vi "Thermopower-v2-SMU1ar-withnVmeter.vi"(0 "Gate Start":dbl format="%#_13g", 1 "hold time (sec)":dbl=10.0 format="%#_13g", 2 "Gate step - extra milliseconds to wait":u32=20000, 4 "N Gate Intervals":i32=7, 5 "Gate Step":dbl=-6.0, 6 "N Heater Intervals":i32=7, 7 "Heater Step":dbl=3.3) -> ()   [LabVIEW 2016]
uses:
  Driver/New driver/Agilent 415X Series.lvlib
  <vilib>/Utility/file.llb/Write To Spreadsheet File (DBL).vi
  <vilib>/Utility/file.llb/Read From Spreadsheet File (DBL).vi
panel:
  out "Voltage across heater (VSU 1 and SMU4) 2":dbl[][](graph)
  out "error out 2":errorcluster
  out "Gate Voltage (SMU 3) 2":dbl[](graph)
  out "Thermal Voltage (SMU2), SMU1 is Common 2":dbl[](graph)
  out "SPA VISA resource name 2":refnum<visa-resource-name>
  out "Voltage across heater (VSU 1 and SMU4)":dbl[][](graph)
  out "Gate Voltage (SMU 3)":dbl[](graph)
  out "Thermal Voltage (SMU2), SMU1 is Common":dbl[](graph)
  in  "SPA VISA resource name":refnum<visa-resource-name>="GPIB0::14::INSTR"
  in  "error in (no error)":errorcluster
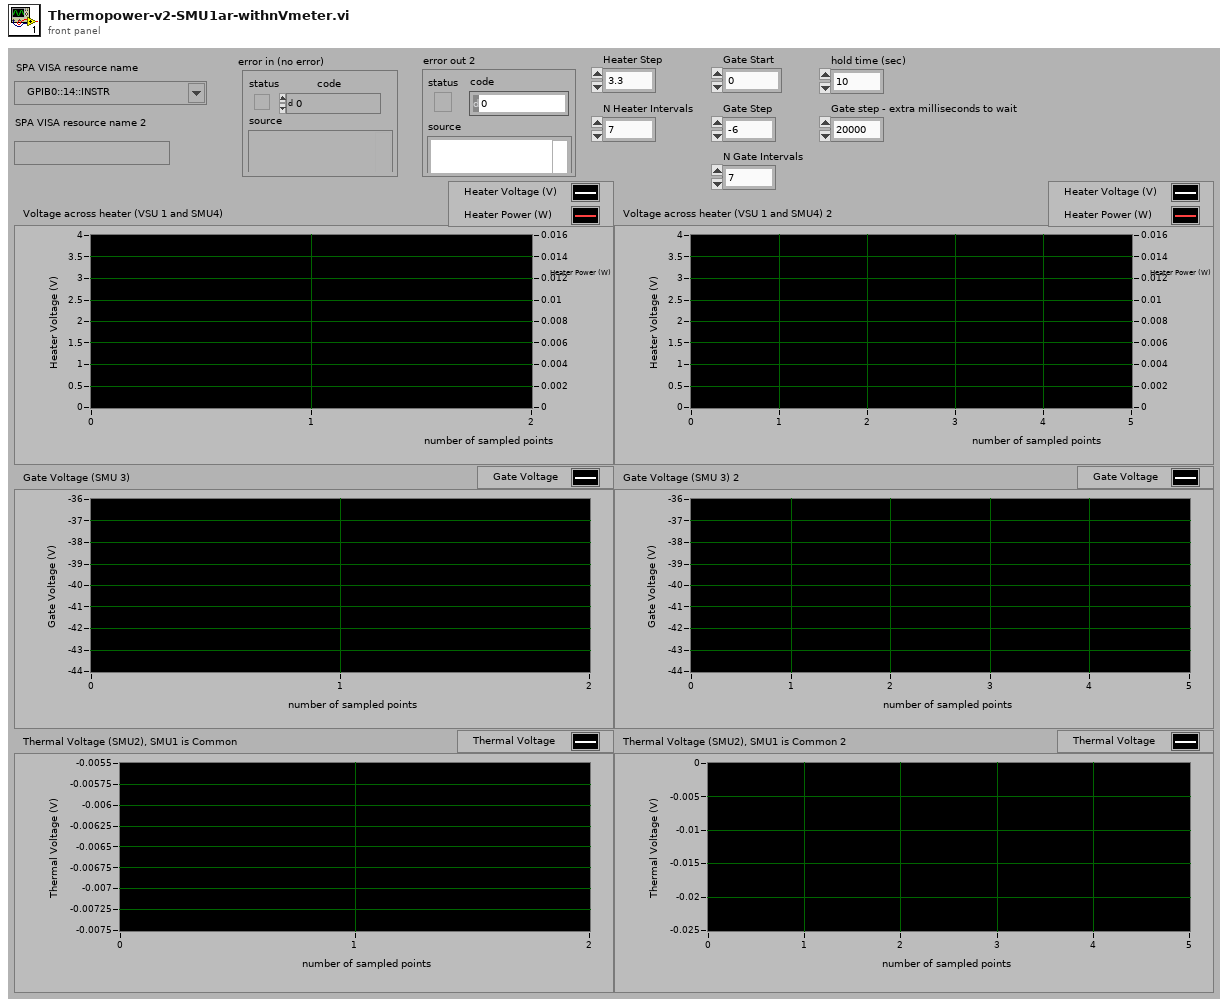
[diagram p1: front panel]
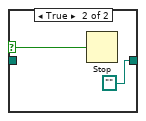
[diagram p3: hidden frame]
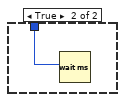
[diagram p4: hidden frame]
diagram:
  # "calculate end gate voltage"
  n1 = flat-sequence {
    tunnel: "error in (no error)" -> [w52]
    tunnel: "SPA VISA resource name" -> [w51]
    tunnel: [w50] -> w45
    tunnel: [w49] -> w44
    tunnel: w45 -> [w59]
    tunnel: w44 -> [w58]
    tunnel: [w55] -> w43
    tunnel: [w54] -> w42
    tunnel: w43 -> [w67]
    tunnel: w42 -> [w66]
    tunnel: [w65] -> w41
    tunnel: [w64] -> w40
    tunnel: w41 -> [w78]
    tunnel: w40 -> [w77]
    tunnel: [w76] -> w39
    tunnel: [w75] -> w38
    tunnel: w39 -> [w89]
    tunnel: w38 -> [w88]
    tunnel: [w87] -> w37
    tunnel: [w86] -> w35
    tunnel: w37 -> [w94]
    tunnel: [w95] -> w36
    tunnel: w35 -> [w93]
    tunnel: [w96] -> w34
    tunnel: w36 -> [w111]
    tunnel: w34 -> [w113]
    tunnel: [w112] -> w27
    tunnel: [w110] -> w26
    tunnel: w27 -> [w115]
    tunnel: w26 -> [w114]
    tunnel: [w118] -> w2
    tunnel: [w117] -> w1
    tunnel: [w128] -> w33
    tunnel: [w131] -> w32
    tunnel: [w130] -> w5
    tunnel: w2 -> [w128]
    tunnel: w1 -> [w129]
    frame #0 {
      n2 = call <instrlib>:"Initialize.vi"("VISA resource name"=refnum<visa-resource-name> "GPIB0::7::INSTR") -> ()  [unwired: 9 in, 2 out]
      n3 = call <instrlib>:"Initialize.vi"("error in (no error)"=w52, "reset"=TRUE, "VISA resource name"=w51) -> ("error out"=w49:errorcluster, "VISA resource name out"=w50:refnum<visa-resource-name>)  [unwired: 2 in, 5 out]
    }
    frame #1 {
      n4 = call "Select-Meas. Mode.vi"("clear all channels"=TRUE, "error in (no error)"=w58, "measurement mode"=TRUE, "VISA resource name"=w59) -> ("error out"=w54:errorcluster, "VISA resource name out"=w55:refnum<visa-resource-name>)  [unwired: 1 in, 5 out]
    }
    frame #2 {
      w62 = 0 items=["0  ", "10K Ohms  ", "100K Ohms  ", "1M Ohms  "] ("series resistance *")
      w63 = 2 items=["V  ", "I  ", "  common  "] ("mode")
      w68 = 0 items=["SMU1  ", "SMU2  ", "SMU3  ", "SMU4  ", "SMU5  ", "SMU6  "] ("unit to configure")
      # "SMU1 configured to be common"
      n5 = call "Config-Chan-SMU-Sampling.vi"("VISA resource name in"=w67, "function"=TRUE, "series resistance *"=w62, "unit to configure"=w68, "V name (max 6 chars)"="Vgnd", "standby"=TRUE, "error in (no error)"=w66, "mode"=w63, "I name (max 6 chars)"="Ignd") -> ("VISA resource name out"=w65:refnum<visa-resource-name>, "error out"=w64:errorcluster)  [unwired: 5 out]
    }
    frame #3 {
      w72 = 0 items=["0  ", "10K Ohms  ", "100K Ohms  ", "1M Ohms  "] ("series resistance *")
      w74 = 1 items=["V  ", "I  ", "  common  "] ("mode")
      w79 = 1 items=["SMU1  ", "SMU2  ", "SMU3  ", "SMU4  ", "SMU5  ", "SMU6  "] ("unit to configure")
      # "SMU2 configured to source current (to be set to zero) \nand measure the thermal voltage"
      n6 = call "Config-Chan-SMU-Sampling.vi"("VISA resource name in"=w78, "function"=TRUE, "series resistance *"=w72, "unit to configure"=w79, "V name (max 6 chars)"="Vth", "standby"=TRUE, "error in (no error)"=w77, "mode"=w74, "I name (max 6 chars)"="Ith") -> ("VISA resource name out"=w76:refnum<visa-resource-name>, "error out"=w75:errorcluster)  [unwired: 5 out]
    }
    frame #4 {
      w83 = 0 items=["0  ", "10K Ohms  ", "100K Ohms  ", "1M Ohms  "] ("series resistance *")
      w85 = 0 items=["V  ", "I  ", "  common  "] ("mode")
      w90 = 2 items=["SMU1  ", "SMU2  ", "SMU3  ", "SMU4  ", "SMU5  ", "SMU6  "] ("unit to configure")
      # "SMU3 configured to source a gate voltage"
      n7 = call "Config-Chan-SMU-Sampling.vi"("VISA resource name in"=w89, "function"=TRUE, "series resistance *"=w83, "unit to configure"=w90, "V name (max 6 chars)"="Vg", "standby"=TRUE, "error in (no error)"=w88, "mode"=w85, "I name (max 6 chars)"="Ig") -> ("VISA resource name out"=w87:refnum<visa-resource-name>, "error out"=w86:errorcluster)  [unwired: 5 out]
    }
    frame #5 {
      w98 = 0 items=["0  ", "10K Ohms  ", "100K Ohms  ", "1M Ohms  "] ("series resistance *")
      w100 = 2 items=["V  ", "I  ", "  common  "] ("mode")
      w101 = 3 items=["SMU1  ", "SMU2  ", "SMU3  ", "SMU4  ", "SMU5  ", "SMU6  "] ("unit to configure")
      # "SMU4 configured to heater ground"
      n8 = call "Config-Chan-SMU-Sampling.vi"("VISA resource name in"=w94, "function"=TRUE, "series resistance *"=w98, "unit to configure"=w101, "V name (max 6 chars)"="Vhgnd", "standby"=TRUE, "error in (no error)"=w93, "mode"=w100, "I name (max 6 chars)"="Ihgnd") -> ("VISA resource name out"=w95:refnum<visa-resource-name>, "error out"=w96:errorcluster)  [unwired: 5 out]
    }
    frame #6 {
      # "VSU1 configured to source a voltage accross a heater"
      n9 = call "Config-Chan-VSUs-Sampling.vi"("VISA session"=w111, "VSU1 function"=TRUE, "VSU2 standby"=TRUE, "VSU1 standby"=FALSE, "VSU1 V name \n(max 6 chars)"="VSU1" ("V name (max 6 chars)"), "VSU2 V name \n(max 6 chars)"="VSU2" ("V name (max 6 chars)"), "error in (no error)"=w113, "VSU2 function"=FALSE) -> ("VISA resource name out"=w110:refnum<visa-resource-name>, "error out"=w112:errorcluster)  [unwired: 6 out]
    }
    frame #7 {
      n10 = VISA Write(VISA resource name=w114, write buffer=":PAGE:MEAS:MSET:SMU2:RANG:MODE FIX", error in (no error)=w115) -> (VISA resource name out=w127:refnum<visa-resource-name>, error out=w126:errorcluster)  [unwired: 1 out]
      n11 = VISA Write(VISA resource name=w127, write buffer=":PAGE:MEAS:MSET:SMU2:RANG 2", error in (no error)=w126) -> (VISA resource name out=w122:refnum<visa-resource-name>, error out=w121:errorcluster)  [unwired: 1 out]
      n12 = VISA Write(VISA resource name=w122, write buffer=":PAGE:MEAS:MSET:ITIM LONG", error in (no error)=w121) -> (VISA resource name out=w120:refnum<visa-resource-name>, error out=w119:errorcluster)  [unwired: 1 out]
      n13 = VISA Write(VISA resource name=w120, write buffer=":PAGE:MEAS:MSET:ITIM:LONG 10", error in (no error)=w119) -> (VISA resource name out=w118:refnum<visa-resource-name>, error out=w117:errorcluster)  [unwired: 1 out]
    }
    frame #8 {
      w130 = 0.0 ("source (V or A)")
      w132 = u16 1 items=["SMU 1", "SMU2", "SMU3", "SMU4", "SMU5", "SMU6", "VSU1", "VSU2"] ("unit (SMU1:0)")
      n14 = call "Config-Sampling-Const-Source.vi"("compliance (SMUs only)"=0.0001, "error in (no error)"=w129, "source (V or A)"=w130, "unit (SMU1:0)"=w132, "VISA session"=w128) -> ("error out"=w131:errorcluster)  [unwired: 6 out]
    }
  }
  n15 = Subtract(x="N Gate Intervals", y=1) -> (x-y=w13:i32)
  n16 = Multiply(x=w13, y="Gate Step") -> (x*y=w11:dbl)
  n17 = Add(x=w11, y="Gate Start") -> (x+y=w10:dbl)
  n18 = call "File Dialog"("start path"=path "C:/users old/khk30", "pattern (all files)"="*.txt") -> ("selected path"=w30:path, "cancelled"=w29:bool)  [unwired: 10 in, 2 out]
  n19 = case shown="False" w29 {
    selector: w29 -> [_ w136]
    tunnel: w30 -> [w134 _]
    tunnel: [w134 path ""] -> w17
    frame False {
    }
    frame True {
      n20 = Stop(stop? (T)=w136) -> ()
    }
  }
  n21 = for {
    N: "N Gate Intervals" -> [_]
    tunnel: w17 -> [w148]
    tunnel: w33 -> [w147]
    tunnel: w32 -> [w146]
    tunnel: [w144] -> w21
    tunnel: [w143] -> w20
    tunnel: "N Heater Intervals" -> [w142]
    tunnel: "Gate Step" -> [w141]
    tunnel: "Gate Start" -> [w140]
    tunnel: "Heater Step" -> [w139]
    tunnel: "Gate step - extra milliseconds to wait" -> [w138]
    tunnel: [w137] -> w6 mode=indexing
    i -> [w145]
    n22 = flat-sequence {
      tunnel: w145 -> [w312]
      tunnel: [w317] -> w150
      tunnel: [w316] -> w149
      tunnel: w147 -> [w315]
      tunnel: w146 -> [w314]
      tunnel: w141 -> [w309]
      tunnel: w140 -> [w308]
      frame #0 {
        w318 = u16 2 items=["SMU 1", "SMU2", "SMU3", "SMU4", "SMU5", "SMU6", "VSU1", "VSU2"] ("unit (SMU1:0)")
        n23 = Multiply(x=w309, y=w312) -> (x*y=w311:dbl)
        n24 = Add(x=w308, y=w311) -> (x+y=w310:dbl)
        n25 = call "Config-Sampling-Const-Source.vi"("compliance (SMUs only)"=0.001, "error in (no error)"=w314, "source (V or A)"=w310, "unit (SMU1:0)"=w318, "VISA session"=w315) -> ("error out"=w316:errorcluster, "VISA resource name out"=w317:refnum<visa-resource-name>)  [unwired: 5 out]
      }
    }
    n26 = for {
      N: w142 -> [_]
      tunnel: w150 -> [w174]
      tunnel: w149 -> [w173]
      tunnel: w148 -> [w172]
      tunnel: w145 -> [w165]
      tunnel: [w160] -> w144
      tunnel: [w159] -> w143
      tunnel: w139 -> [w158]
      tunnel: w138 -> [w157]
      tunnel: [w156] -> w137 mode=indexing
      i -> [w175]
      n27 = flat-sequence {
        tunnel: [w190] -> w183
        tunnel: [w189] -> w182
        tunnel: w175 -> [w185]
        tunnel: w174 -> [w188]
        tunnel: w173 -> [w187]
        tunnel: [w185] -> w166
        tunnel: w158 -> [w184]
        tunnel: w183 -> [w200]
        tunnel: w182 -> [w198]
        tunnel: [w199] -> w181
        tunnel: [w198] -> w180
        tunnel: w166 -> [w194]
        tunnel: w165 -> [w193]
        tunnel: w157 -> [w192]
        tunnel: w181 -> [w207]
        tunnel: w180 -> [w206]
        tunnel: [w205] -> w179
        tunnel: [w204] -> w178
        tunnel: ["hold time (sec)"] -> w156
        tunnel: w179 -> [w217]
        tunnel: w178 -> [w216]
        tunnel: [w215] -> w177
        tunnel: [w214] -> w176
        tunnel: w177 -> [w223]
        tunnel: w176 -> [w222]
        tunnel: [w221] -> w155
        tunnel: [w220] -> w153
        tunnel: w155 -> [w234]
        tunnel: [w234] -> w154
        tunnel: w153 -> [w233]
        tunnel: [w233] -> w152
        tunnel: [w227] -> w151
        tunnel: w154 -> [w251]
        tunnel: w152 -> [w250]
        tunnel: w172 -> [w252]
        tunnel: [w252] -> w171
        tunnel: [w252] -> w170
        tunnel: [w238] -> w168
        tunnel: [w240] -> w160
        tunnel: w151 -> [w235]
        tunnel: w171 -> [w279]
        tunnel: [w277] -> w164
        tunnel: w170 -> [w277]
        tunnel: w168 -> [w274]
        tunnel: [w274] -> w162
        tunnel: w164 -> [w283]
        tunnel: [w283] -> w163
        tunnel: w162 -> [w284]
        tunnel: [w284] -> w161
        tunnel: w163 -> [w289]
        tunnel: [w289] -> w169
        tunnel: w161 -> [w285]
        tunnel: [w285] -> w167
        tunnel: w169 -> [w303]
        tunnel: w167 -> [w294]
        tunnel: [w294] -> w159
        frame #0 {
          w191 = u16 6 items=["SMU 1", "SMU2", "SMU3", "SMU4", "SMU5", "SMU6", "VSU1", "VSU2"] ("unit (SMU1:0)")
          n28 = Multiply(x=w184, y=w185) -> (x*y=w186:dbl)
          n29 = call "Config-Sampling-Const-Source.vi"("error in (no error)"=w187, "source (V or A)"=w186, "unit (SMU1:0)"=w191, "VISA session"=w188) -> ("error out"=w190:errorcluster, "VISA resource name out"=w189:refnum<visa-resource-name>)  [unwired: 1 in, 5 out]
        }
        frame #1 {
          n30 = Equal To 0?(x=w194) -> (x = 0?=w195:bool)
          n31 = Greater Than 0?(x=w193) -> (x > 0?=w196:bool)
          n32 = And(x=w195, y=w196) -> (x .and. y?=w197:bool)
          n33 = call "Config-Display-List.vi"("error in (no error)"=w200, "list (max 8 elements)"=string[] ["Vth", "Ith", "VSU1", "Ihgnd", "Vg", "Ig", "Ignd"], "VISA session"=w198) -> ("error out"=w199:errorcluster)  [unwired: 1 in, 7 out]
          n34 = case shown="False" w197 {
            tunnel: w192 -> [_ w202]
            frame False {
            }
            frame True {
              n35 = Wait (ms)(milliseconds to wait=w202) -> ()  [unwired: 1 out]
            }
          }
        }
        frame #2 {
          w208 = 100.0  # sampling time limit
          w209 = 0 items=["linear", "log 10", "log 25", "log 50", "thinned out"] ("mode (linear: 0)")
          w210 = 0 items=["auto (linear only)", "no limit", "set limit "] ("sampling time\n(linear/thinned-out only)")
          w211 = 0.1  # initial interval (sec)
          w212 = 10  # num. of events
          w213 = 1  # number of samples
          n36 = call "Config-Sampling-Parameters.vi"("VISA session"=w206, "mode (linear: 0)"=w209, "initial interval (sec)"=w211, "sampling time\n(linear/thinned-out only)"=w210, "number of samples"=w213, "error in (no error)"=w207, "sampling time limit"=w208, "num. of events"=w212, "hold time (sec)"="hold time (sec)") -> ("VISA resource name out"=w204:refnum<visa-resource-name>, "error out"=w205:errorcluster)  [unwired: 7 in, 10 out]
        }
        frame #3 {
          w219 = 2 items=["short  ", "medium  ", "long  "] ("integration time")
          n37 = call "Config-Meas-Timing.vi"("# PLCs for long integration time"=1, "error in (no error)"=w217, "integration time"=w219, "VISA session"=w216) -> ("error out"=w215:errorcluster, "VISA resource name out"=w214:refnum<visa-resource-name>)  [unwired: 2 in, 4 out]
        }
        frame #4 {
          w225 = 1 items=["stop  ", "single  ", "single-append  ", "stress start  ", "continuous  ", "standby on  ", "standby off  ", "zero  "] ("function (stop:0)")
          n38 = call "Op-Start-Stop.vi"("time to wait (30000ms)"=600000, "error in (no error)"=w223, "function (stop:0)"=w225, "wait until finish"=TRUE, "VISA resource name"=w222) -> ("error out"=w221:errorcluster, "VISA resource name out"=w220:refnum<visa-resource-name>)  [unwired: 5 out]
        }
        frame #5 {
          n39 = call "READ.vi"("VISA resource name"=refnum<visa-resource-name> "GPIB0::7::INSTR") -> ("read buffer"=w232:string)  [unwired: 9 in, 1 out]
          n40 = Fract/Exp String To Number(string=w232) -> (number=w228:dbl)  [unwired: 3 in, 1 out]
          n41 = Build Array(0.0) -> (w229:dbl[])
          n42 = Type Cast(type=w229, x=w228) -> (*(type *) &x=w227:dbl[])
        }
        frame #6 {
          # "Computes Heater power via P=VI"
          n43 = call "4155C DOWNLOAD variable.vi"("error in (no error)"=w251, "Variable name"="Vth", "VISA resource name in"=w250) -> ("error out"=w259:errorcluster, "Output data"=w246:dbl[], "VISA Resource Name out"=w264:refnum<visa-resource-name>)  [unwired: 2 out]
          n44 = call "4155C DOWNLOAD variable.vi"("error in (no error)"=w259, "Variable name"="Ith", "VISA resource name in"=w264) -> ("error out"=w258:errorcluster, "Output data"=w247:dbl[], "VISA Resource Name out"=w263:refnum<visa-resource-name>)  [unwired: 2 out]
          n45 = call "4155C DOWNLOAD variable.vi"("error in (no error)"=w258, "Variable name"="VSU1", "VISA resource name in"=w263) -> ("error out"=w257:errorcluster, "Output data"=w244:dbl[], "VISA Resource Name out"=w262:refnum<visa-resource-name>)  [unwired: 2 out]
          n46 = call "4155C DOWNLOAD variable.vi"("error in (no error)"=w257, "Variable name"="Ihgnd", "VISA resource name in"=w262) -> ("error out"=w256:errorcluster, "Output data"=w245:dbl[], "VISA Resource Name out"=w261:refnum<visa-resource-name>)  [unwired: 2 out]
          n47 = Multiply(x=w244, y=w245) -> (x*y=w249:dbl[])
          n48 = Absolute Value(x=w249) -> (abs(x)=w243:dbl[])
          n49 = call "4155C DOWNLOAD variable.vi"("error in (no error)"=w256, "Variable name"="Vg", "VISA resource name in"=w261) -> ("error out"=w255:errorcluster, "Output data"=w248:dbl[], "VISA Resource Name out"=w260:refnum<visa-resource-name>)  [unwired: 2 out]
          n50 = call "4155C DOWNLOAD variable.vi"("error in (no error)"=w255, "Variable name"="Ig", "VISA resource name in"=w260) -> ("error out"=w239:errorcluster, "Output data"=w237:dbl[], "VISA Resource Name out"=w242:refnum<visa-resource-name>)  [unwired: 2 out]
          n51 = call "4155C DOWNLOAD variable.vi"("error in (no error)"=w239, "Variable name"="Ignd", "VISA resource name in"=w242) -> ("error out"=w238:errorcluster, "Output data"=w236:dbl[], "VISA Resource Name out"=w240:refnum<visa-resource-name>)  [unwired: 2 out]
          n52 = Build Array(w243, w244, w245, w246, w247, w248, w237, w236, w235) -> (w254:dbl[][])
          n53 = call-poly <vilib>:"Write To Spreadsheet File.vi"("transpose? (no:F)"=TRUE, "format (%.3f)"="%.13f", "append to file? (new file:F)"=TRUE, "2D data"=w254, "file path (dialog if empty)"=w252) -> ()  [unwired: 1 in, 3 out]
        }
        frame #7 {
          # "plot the thermal voltage after reading the file"
          n54 = call-poly <vilib>:"Read From Spreadsheet File.vi"("transpose (no:F)"=TRUE, "format (%.3f)"="%.13f", "max characters/row  (no limit:0)"=0, "number of rows (all:-1)"=-1, "file path (dialog if empty)"=w279) -> ("all rows"=w276:dbl[][])  [unwired: 6 out]
          n55 = Index Array(array=w276, index (row)=8) -> (element=→"Thermal Voltage (SMU2), SMU1 is Common":dbl[])  [unwired: 1 in]
        }
        frame #8 {
        }
        frame #9 {
          # "plot the gate voltage after reading the file"
          n56 = call-poly <vilib>:"Read From Spreadsheet File.vi"("transpose (no:F)"=TRUE, "format (%.3f)"="%.13f", "max characters/row  (no limit:0)"=0, "number of rows (all:-1)"=-1, "file path (dialog if empty)"=w289) -> ("all rows"=w288:dbl[][])  [unwired: 6 out]
          n57 = Index Array(array=w288, index (row)=5) -> (element=→"Gate Voltage (SMU 3)":dbl[])  [unwired: 1 in]
        }
        frame #10 {
          # "plot the voltage across the heater and the \npower dissipated by the heater after reading the file"
          n58 = call-poly <vilib>:"Read From Spreadsheet File.vi"("transpose (no:F)"=TRUE, "format (%.3f)"="%.13f", "max characters/row  (no limit:0)"=0, "number of rows (all:-1)"=-1, "file path (dialog if empty)"=w303) -> ("all rows"=w301:dbl[][])  [unwired: 6 out]
          n59 = Index Array(array=w301, index (row)=1) -> (element=w295:dbl[])  [unwired: 1 in]
          n60 = Index Array(array=w301, index (row)=2) -> (element=w299:dbl[])  [unwired: 1 in]
          n61 = Multiply(x=w295, y=w299) -> (x*y=w298:dbl[])
          n62 = Absolute Value(x=w298) -> (abs(x)=w297:dbl[])
          n63 = Build Array(w295, w297) -> (→"Voltage across heater (VSU 1 and SMU4)":dbl[][])
        }
      }
    }
  }
  n64 = flat-sequence {
    tunnel: [w326] -> w25
    tunnel: [w325] -> w24
    tunnel: w21 -> [w320]
    tunnel: w20 -> [w319]
    tunnel: w25 -> [w337]
    tunnel: w24 -> [w336]
    tunnel: [w331] -> w4
    tunnel: [w330] -> w3
    tunnel: [w341] -> w23
    tunnel: [w342] -> w22
    tunnel: w4 -> [w344]
    tunnel: w3 -> [w343]
    tunnel: w23 -> [w352]
    tunnel: w22 -> [w353]
    tunnel: [w351] -> w18
    tunnel: [w350] -> w19
    tunnel: w5 -> [w349]
    frame #0 {
      w323 = 0 items=["0  ", "10K Ohms  ", "100K Ohms  ", "1M Ohms  "] ("series resistance *")
      w324 = 2 items=["V  ", "I  ", "  common  "] ("mode")
      w327 = 1 items=["SMU1  ", "SMU2  ", "SMU3  ", "SMU4  ", "SMU5  ", "SMU6  "] ("unit to configure")
      # "SMU2 configured to be common"
      n65 = call "Config-Chan-SMU-Sampling.vi"("VISA resource name in"=w320, "function"=TRUE, "series resistance *"=w323, "unit to configure"=w327, "V name (max 6 chars)"="Vgnd", "standby"=TRUE, "error in (no error)"=w319, "mode"=w324, "I name (max 6 chars)"="Ignd") -> ("VISA resource name out"=w326:refnum<visa-resource-name>, "error out"=w325:errorcluster)  [unwired: 5 out]
    }
    frame #1 {
      w333 = 0 items=["0  ", "10K Ohms  ", "100K Ohms  ", "1M Ohms  "] ("series resistance *")
      w335 = 1 items=["V  ", "I  ", "  common  "] ("mode")
      w338 = 0 items=["SMU1  ", "SMU2  ", "SMU3  ", "SMU4  ", "SMU5  ", "SMU6  "] ("unit to configure")
      # "SMU2 configured to source current (to be set to zero) \nand measure the thermal voltage"
      n66 = call "Config-Chan-SMU-Sampling.vi"("VISA resource name in"=w337, "function"=TRUE, "series resistance *"=w333, "unit to configure"=w338, "V name (max 6 chars)"="Vth", "standby"=TRUE, "error in (no error)"=w336, "mode"=w335, "I name (max 6 chars)"="Ith") -> ("VISA resource name out"=w331:refnum<visa-resource-name>, "error out"=w330:errorcluster)  [unwired: 5 out]
    }
    frame #2 {
      n67 = VISA Write(VISA resource name=w344, write buffer=":PAGE:MEAS:MSET:SMU1:RANG:MODE FIX", error in (no error)=w343) -> (VISA resource name out=w347:refnum<visa-resource-name>, error out=w346:errorcluster)  [unwired: 1 out]
      n68 = VISA Write(VISA resource name=w347, write buffer=":PAGE:MEAS:MSET:SMU1:RANG 2", error in (no error)=w346) -> (VISA resource name out=w342:refnum<visa-resource-name>, error out=w341:errorcluster)  [unwired: 1 out]
    }
    frame #3 {
      w354 = u16 0 items=["SMU 1", "SMU2", "SMU3", "SMU4", "SMU5", "SMU6", "VSU1", "VSU2"] ("unit (SMU1:0)")
      n69 = call "Config-Sampling-Const-Source.vi"("compliance (SMUs only)"=0.0001, "error in (no error)"=w352, "source (V or A)"=w349, "unit (SMU1:0)"=w354, "VISA session"=w353) -> ("error out"=w350:errorcluster, "VISA resource name out"=w351:refnum<visa-resource-name>)  [unwired: 5 out]
    }
  }
  n70 = for {
    N: "N Gate Intervals" -> [_]
    tunnel: w17 -> [w367]
    tunnel: w18 -> [w366]
    tunnel: w19 -> [w365]
    tunnel: [w363] -> _
    tunnel: [w362] -> _
    tunnel: "N Heater Intervals" -> [w361]
    tunnel: w10 -> [w360]
    tunnel: "Gate Step" -> [w359]
    tunnel: "Heater Step" -> [w358]
    tunnel: "Gate step - extra milliseconds to wait" -> [w357]
    tunnel: w6 -> [w356] mode=indexing
    i -> [w364]
    n71 = flat-sequence {
      tunnel: w364 -> [w536]
      tunnel: [w541] -> w369
      tunnel: [w540] -> w368
      tunnel: w366 -> [w539]
      tunnel: w365 -> [w538]
      tunnel: w360 -> [w534]
      tunnel: w359 -> [w532]
      frame #0 {
        w542 = u16 2 items=["SMU 1", "SMU2", "SMU3", "SMU4", "SMU5", "SMU6", "VSU1", "VSU2"] ("unit (SMU1:0)")
        n72 = Multiply(x=w532, y=w536) -> (x*y=w533:dbl)
        n73 = Subtract(x=w534, y=w533) -> (x-y=w535:dbl)
        n74 = call "Config-Sampling-Const-Source.vi"("compliance (SMUs only)"=0.001, "error in (no error)"=w538, "source (V or A)"=w535, "unit (SMU1:0)"=w542, "VISA session"=w539) -> ("error out"=w540:errorcluster, "VISA resource name out"=w541:refnum<visa-resource-name>)  [unwired: 5 out]
      }
    }
    n75 = for {
      N: w361 -> [_]
      tunnel: w369 -> [w393]
      tunnel: w368 -> [w392]
      tunnel: w367 -> [w391]
      tunnel: w364 -> [w384]
      tunnel: [w379] -> w363
      tunnel: [w378] -> w362
      tunnel: w358 -> [w377]
      tunnel: w357 -> [w376]
      tunnel: w356 -> [w375] mode=indexing
      i -> [w394]
      n76 = flat-sequence {
        tunnel: [w409] -> w402
        tunnel: [w408] -> w401
        tunnel: w394 -> [w404]
        tunnel: w393 -> [w407]
        tunnel: w392 -> [w406]
        tunnel: [w404] -> w385
        tunnel: w377 -> [w403]
        tunnel: w402 -> [w419]
        tunnel: w401 -> [w417]
        tunnel: [w418] -> w400
        tunnel: [w417] -> w399
        tunnel: w385 -> [w413]
        tunnel: w384 -> [w412]
        tunnel: w376 -> [w411]
        tunnel: w400 -> [w426]
        tunnel: w399 -> [w425]
        tunnel: [w424] -> w398
        tunnel: [w423] -> w397
        tunnel: w375 -> [w422]
        tunnel: w398 -> [w436]
        tunnel: w397 -> [w435]
        tunnel: [w434] -> w396
        tunnel: [w433] -> w395
        tunnel: w396 -> [w442]
        tunnel: w395 -> [w441]
        tunnel: [w440] -> w374
        tunnel: [w439] -> w372
        tunnel: w374 -> [w453]
        tunnel: [w453] -> w373
        tunnel: w372 -> [w452]
        tunnel: [w452] -> w371
        tunnel: [w446] -> w370
        tunnel: w373 -> [w470]
        tunnel: w371 -> [w469]
        tunnel: w391 -> [w471]
        tunnel: [w471] -> w390
        tunnel: [w471] -> w389
        tunnel: [w458] -> w387
        tunnel: [w457] -> w379
        tunnel: w370 -> [w454]
        tunnel: w390 -> [w498]
        tunnel: [w496] -> w383
        tunnel: w389 -> [w496]
        tunnel: w387 -> [w493]
        tunnel: [w493] -> w381
        tunnel: w383 -> [w502]
        tunnel: [w502] -> w382
        tunnel: w381 -> [w503]
        tunnel: [w503] -> w380
        tunnel: w382 -> [w508]
        tunnel: [w508] -> w388
        tunnel: w380 -> [w504]
        tunnel: [w504] -> w386
        tunnel: w388 -> [w527]
        tunnel: w386 -> [w513]
        tunnel: [w513] -> w378
        frame #0 {
          w410 = u16 6 items=["SMU 1", "SMU2", "SMU3", "SMU4", "SMU5", "SMU6", "VSU1", "VSU2"] ("unit (SMU1:0)")
          n77 = Multiply(x=w403, y=w404) -> (x*y=w405:dbl)
          n78 = call "Config-Sampling-Const-Source.vi"("error in (no error)"=w406, "source (V or A)"=w405, "unit (SMU1:0)"=w410, "VISA session"=w407) -> ("error out"=w409:errorcluster, "VISA resource name out"=w408:refnum<visa-resource-name>)  [unwired: 1 in, 5 out]
        }
        frame #1 {
          n79 = Equal To 0?(x=w413) -> (x = 0?=w414:bool)
          n80 = Greater Than 0?(x=w412) -> (x > 0?=w415:bool)
          n81 = And(x=w414, y=w415) -> (x .and. y?=w416:bool)
          n82 = call "Config-Display-List.vi"("error in (no error)"=w419, "list (max 8 elements)"=string[] ["Vth", "Ith", "VSU1", "Ihgnd", "Vg", "Ig", "Ignd"], "VISA session"=w417) -> ("error out"=w418:errorcluster)  [unwired: 1 in, 7 out]
          n83 = case shown="True" w416 {
            tunnel: w411 -> [_ w421]
            frame False {
            }
            frame True {
              n84 = Wait (ms)(milliseconds to wait=w421) -> ()  [unwired: 1 out]
            }
          }
        }
        frame #2 {
          w427 = 100.0  # sampling time limit
          w428 = 0 items=["linear", "log 10", "log 25", "log 50", "thinned out"] ("mode (linear: 0)")
          w429 = 0 items=["auto (linear only)", "no limit", "set limit "] ("sampling time\n(linear/thinned-out only)")
          w430 = 0.1  # initial interval (sec)
          w431 = 10  # num. of events
          w432 = 1  # number of samples
          n85 = call "Config-Sampling-Parameters.vi"("VISA session"=w425, "mode (linear: 0)"=w428, "initial interval (sec)"=w430, "sampling time\n(linear/thinned-out only)"=w429, "number of samples"=w432, "error in (no error)"=w426, "sampling time limit"=w427, "num. of events"=w431, "hold time (sec)"=w422) -> ("VISA resource name out"=w423:refnum<visa-resource-name>, "error out"=w424:errorcluster)  [unwired: 7 in, 10 out]
        }
        frame #3 {
          w438 = 2 items=["short  ", "medium  ", "long  "] ("integration time")
          n86 = call "Config-Meas-Timing.vi"("# PLCs for long integration time"=1, "error in (no error)"=w436, "integration time"=w438, "VISA session"=w435) -> ("error out"=w434:errorcluster, "VISA resource name out"=w433:refnum<visa-resource-name>)  [unwired: 2 in, 4 out]
        }
        frame #4 {
          w444 = 1 items=["stop  ", "single  ", "single-append  ", "stress start  ", "continuous  ", "standby on  ", "standby off  ", "zero  "] ("function (stop:0)")
          n87 = call "Op-Start-Stop.vi"("time to wait (30000ms)"=600000, "error in (no error)"=w442, "function (stop:0)"=w444, "wait until finish"=TRUE, "VISA resource name"=w441) -> ("error out"=w440:errorcluster, "VISA resource name out"=w439:refnum<visa-resource-name>)  [unwired: 5 out]
        }
        frame #5 {
          n88 = call "READ.vi"("VISA resource name"=refnum<visa-resource-name> "GPIB0::7::INSTR") -> ("read buffer"=w450:string)  [unwired: 9 in, 1 out]
          n89 = Build Array(0.0) -> (w449:dbl[])
          n90 = Fract/Exp String To Number(string=w450) -> (number=w447:dbl)  [unwired: 3 in, 1 out]
          n91 = Type Cast(type=w449, x=w447) -> (*(type *) &x=w446:dbl[])
        }
        frame #6 {
          # "Computes Heater power via P=VI"
          n92 = call "4155C DOWNLOAD variable.vi"("error in (no error)"=w470, "Variable name"="Vth", "VISA resource name in"=w469) -> ("error out"=w478:errorcluster, "Output data"=w464:dbl[], "VISA Resource Name out"=w483:refnum<visa-resource-name>)  [unwired: 2 out]
          n93 = call "4155C DOWNLOAD variable.vi"("error in (no error)"=w478, "Variable name"="Ith", "VISA resource name in"=w483) -> ("error out"=w477:errorcluster, "Output data"=w465:dbl[], "VISA Resource Name out"=w482:refnum<visa-resource-name>)  [unwired: 2 out]
          n94 = call "4155C DOWNLOAD variable.vi"("error in (no error)"=w477, "Variable name"="VSU1", "VISA resource name in"=w482) -> ("error out"=w476:errorcluster, "Output data"=w462:dbl[], "VISA Resource Name out"=w481:refnum<visa-resource-name>)  [unwired: 2 out]
          n95 = call "4155C DOWNLOAD variable.vi"("error in (no error)"=w476, "Variable name"="Ihgnd", "VISA resource name in"=w481) -> ("error out"=w475:errorcluster, "Output data"=w463:dbl[], "VISA Resource Name out"=w480:refnum<visa-resource-name>)  [unwired: 2 out]
          n96 = Multiply(x=w462, y=w463) -> (x*y=w468:dbl[])
          n97 = Absolute Value(x=w468) -> (abs(x)=w461:dbl[])
          n98 = call "4155C DOWNLOAD variable.vi"("error in (no error)"=w475, "Variable name"="Vg", "VISA resource name in"=w480) -> ("error out"=w474:errorcluster, "Output data"=w466:dbl[], "VISA Resource Name out"=w479:refnum<visa-resource-name>)  [unwired: 2 out]
          n99 = call "4155C DOWNLOAD variable.vi"("error in (no error)"=w474, "Variable name"="Ig", "VISA resource name in"=w479) -> ("error out"=w459:errorcluster, "Output data"=w467:dbl[], "VISA Resource Name out"=w460:refnum<visa-resource-name>)  [unwired: 2 out]
          n100 = call "4155C DOWNLOAD variable.vi"("error in (no error)"=w459, "Variable name"="Ignd", "VISA resource name in"=w460) -> ("error out"=w458:errorcluster, "Output data"=w456:dbl[], "VISA Resource Name out"=w457:refnum<visa-resource-name>)  [unwired: 2 out]
          "SPA VISA resource name 2" <- w457
          n101 = Build Array(w461, w462, w463, w464, w465, w466, w467, w456, w454) -> (w473:dbl[][])
          n102 = call-poly <vilib>:"Write To Spreadsheet File.vi"("transpose? (no:F)"=TRUE, "format (%.3f)"="%.13f", "append to file? (new file:F)"=TRUE, "2D data"=w473, "file path (dialog if empty)"=w471) -> ()  [unwired: 1 in, 3 out]
        }
        frame #7 {
          # "plot the thermal voltage after reading the file"
          n103 = call-poly <vilib>:"Read From Spreadsheet File.vi"("transpose (no:F)"=TRUE, "format (%.3f)"="%.13f", "max characters/row  (no limit:0)"=0, "number of rows (all:-1)"=-1, "file path (dialog if empty)"=w498) -> ("all rows"=w495:dbl[][])  [unwired: 6 out]
          n104 = Index Array(array=w495, index (row)=8) -> (element=→"Thermal Voltage (SMU2), SMU1 is Common 2":dbl[])  [unwired: 1 in]
        }
        frame #8 {
        }
        frame #9 {
          # "plot the gate voltage after reading the file"
          n105 = call-poly <vilib>:"Read From Spreadsheet File.vi"("transpose (no:F)"=TRUE, "format (%.3f)"="%.13f", "max characters/row  (no limit:0)"=0, "number of rows (all:-1)"=-1, "file path (dialog if empty)"=w508) -> ("all rows"=w507:dbl[][])  [unwired: 6 out]
          n106 = Index Array(array=w507, index (row)=5) -> (element=→"Gate Voltage (SMU 3) 2":dbl[])  [unwired: 1 in]
        }
        frame #10 {
          # "plot the voltage across the heater and the \npower dissipated by the heater after reading the file"
          n107 = call-poly <vilib>:"Read From Spreadsheet File.vi"("transpose (no:F)"=TRUE, "format (%.3f)"="%.13f", "max characters/row  (no limit:0)"=0, "number of rows (all:-1)"=-1, "file path (dialog if empty)"=w527) -> ("all rows"=w525:dbl[][])  [unwired: 6 out]
          n108 = Index Array(array=w525, index (row)=1) -> (element=w519:dbl[])  [unwired: 1 in]
          n109 = Index Array(array=w525, index (row)=2) -> (element=w523:dbl[])  [unwired: 1 in]
          n110 = property on="Voltage across heater (VSU 1 and SMU4) 2" class="WFGraph (strict)"(error in=w513, "Active Plot"=u32 0, "Plot.YScaleIdx"=u32 0 ("Plot.Y Scale Index"), "Active Plot"=u32 1, "Plot.YScaleIdx"=u32 1 ("Plot.Y Scale Index")) -> (error out=→"error out 2":errorcluster)  [unwired: 1 in, 1 out]
          n111 = Multiply(x=w519, y=w523) -> (x*y=w522:dbl[])
          n112 = Absolute Value(x=w522) -> (abs(x)=w521:dbl[])
          n113 = Build Array(w519, w521) -> (→"Voltage across heater (VSU 1 and SMU4) 2":dbl[][])
        }
      }
    }
  }
